vi "Convert Server Topic Filter Matching.vi"(8 "error in (no error)":errorcluster, 10 "Matching Topic Filter":string, 11 "PUBLISH":refnum<class "PUBLISH.lvclass">) -> (0 "error out":errorcluster, 3 "Server PUBLISH":refnum<class "PUBLISH.lvclass">)   [LabVIEW 2013, in "PUBLISH.lvclass"]
uses:
  PUBLISH.lvclass
  ControlPacket/ControlPacket.lvclass/ControlPacket.ctl
  PUBLISH.lvclass/PUBLISH.ctl
  ControlPacket/ControlPacket.lvclass
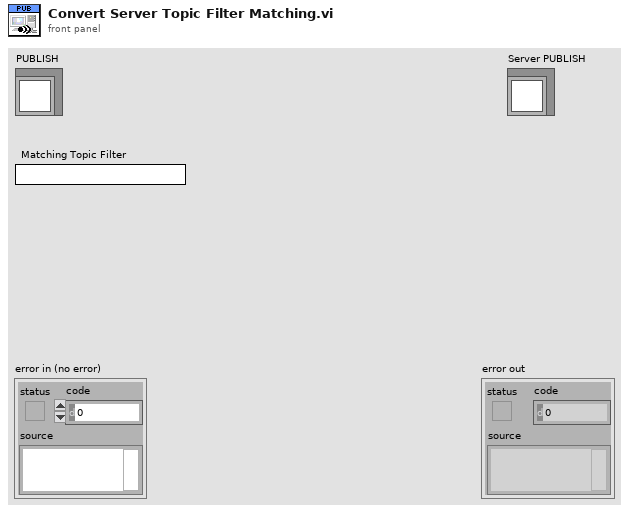
[diagram p1: front panel]
types:
  T1 = typedef "ControlPacket.lvclass/QualityOfService -- enum.ctl" = enum16{"0 (At Most Once)", "1 (At Least Once)", "2 (Exactly Once)"}
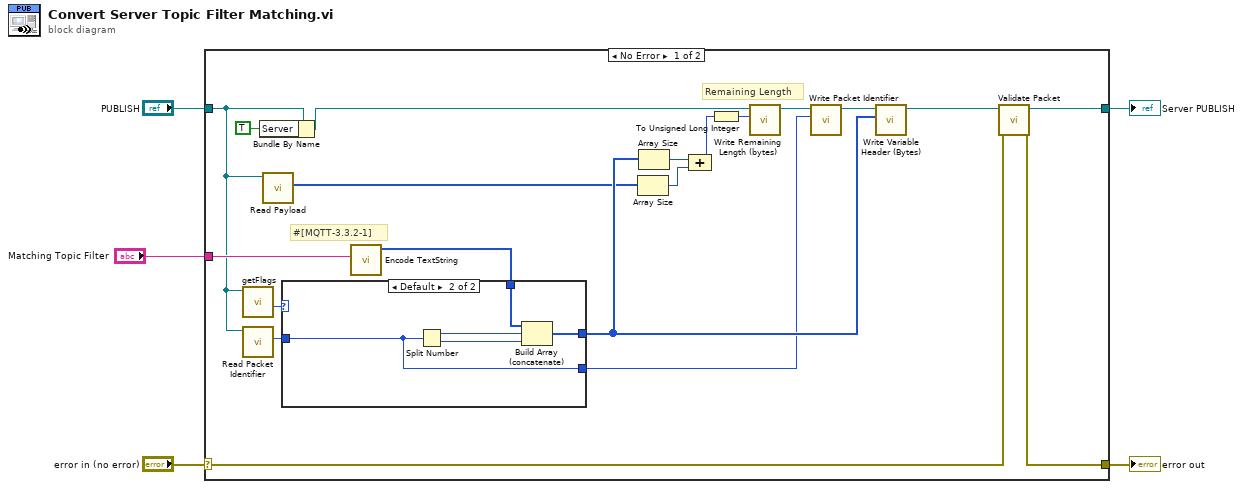
[diagram p0: block diagram]
diagram:
  n1 = case shown="No Error" "error in (no error)" {
    selector: "error in (no error)" -> [w14 w33]
    tunnel: [w13 w33] -> w4
    tunnel: [w15 w32] -> w2
    tunnel: "PUBLISH" -> [w8 w32]
    tunnel: "Matching Topic Filter" -> [w25 _]
    frame No Error {
      # "#[MQTT-3.3.2-1]"
      # "Remaining Length"
      n2 = call-dynamic "getFlags.vi"("PUBLISH in"=w8) -> ("QoS"=w9:T1)  [unwired: 7 in, 3 out]
      n3 = call "Read Packet Identifier.vi"("ControlPacket in"=w8) -> ("Packet Identifier"=w10:u16)  [unwired: 9 in, 1 out]
      n4 = Bundle By Name(cluster=w8, "Server"=TRUE) -> (w6:refnum<class "PUBLISH.lvclass">)
      n5 = call "Read Payload.vi"("ControlPacket in"=w8) -> ("Payload"=w7:u8[])  [unwired: 9 in, 1 out]
      n6 = call "Encode TextString.vi"("Text String"=w25) -> ("Length-Prefixed Field"=w23:u8[])  [unwired: 10 in]
      n7 = case shown="Default" w9 {
        tunnel: w23 -> [w26 w31]
        tunnel: [w26 w28] -> w22
        tunnel: w10 -> [_ w27]
        tunnel: [_ w27] -> w16
        frame "0 (At Most Once)" {
          # "#[MQTT-2.3.1-5]"
        }
        frame Default {
          n8 = Split Number(x=w27) -> (hi(x)=w30:u8, lo(x)=w29:u8)
          n9 = Build Array (concatenate)(w31, w30, w29) -> (w28:u8[])
        }
      }
      n10 = Array Size(array=w7) -> (size(s)=w20:i32)
      n11 = Array Size(array=w22) -> (size(s)=w21:i32)
      n12 = Compound Arithmetic op=ADD(w21, w20) -> (w19:i32)
      n13 = To Unsigned Long Integer(number=w19) -> (unsigned 32bit integer=w24:u32)
      n14 = call "Write Remaining Length (bytes).vi"("Remaining Length (bytes)"=w24, "ControlPacket in"=w6) -> ("ControlPacket out"=w18:refnum<class "PUBLISH.lvclass">)  [unwired: 9 in]
      n15 = call "Write Packet Identifier.vi"("Packet Identifier"=w16, "ControlPacket in"=w18) -> ("ControlPacket out"=w17:refnum<class "PUBLISH.lvclass">)  [unwired: 9 in]
      n16 = call "Write Variable Header (Bytes).vi"("Variable Header (Bytes)"=w22, "ControlPacket in"=w17) -> ("ControlPacket out"=w11:refnum<class "PUBLISH.lvclass">)  [unwired: 9 in]
      n17 = call "Validate Packet.vi"("error in (no error)"=w14, "ControlPacket in"=w11) -> ("error out"=w13:errorcluster, "ControlPacket out"=w15:refnum<class "PUBLISH.lvclass">)  [unwired: 8 in]
    }
    frame Error {
    }
  }
  "error out" <- w4
  "Server PUBLISH" <- w2
